vi "CRYGet Current HC Steps.vi"() -> (2 "Calibration setup flattened Out":string, 3 "Hardware setup flattened Out":string)   [LabVIEW 2013]
uses:
  CRYProject Editor Global.vi
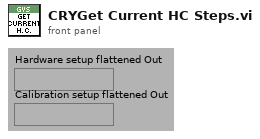
[diagram p1: front panel]
types:
  T1 = typedef "CRYStep.ctl" = cluster{"No.VI":i32, "Category":string, "StepName":string, "Seq setup flattened":string, "Comment":string, "Steps config.":bool[], "Jump config":i32[], "Start":dbl, "Increment":dbl, "Name":string, "Unit":string, "Y data":u16, "Y prefix":string, "Y dB ref":dbl, "Y unit":string, "Repeat State Array":cluster{"Start":dbl, "Increment":dbl, "Count":i32, "Num":i32}[]}
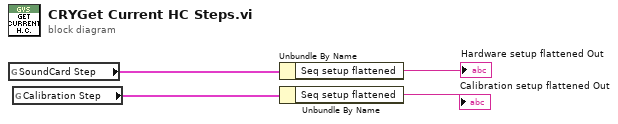
[diagram p0: block diagram]
diagram:
  n1 = global read "CRYProject Editor Global.vi" "SoundCard Step"() -> (w4:T1)
  n2 = global read "CRYProject Editor Global.vi" "Calibration Step"() -> (w3:T1)
  n3 = Unbundle By Name(w4) -> ("Seq setup flattened"=→"Hardware setup flattened Out":string)
  n4 = Unbundle By Name(w3) -> ("Seq setup flattened"=→"Calibration setup flattened Out":string)
